vi "AllVIs.vi"   [LabVIEW 2023]
doc: "This VI hosts the full list of Redis in LabVIEW developed VIs."
uses:
  Palette/Redis Commands/Connection/AUTH.vi
  Palette/Redis Commands/Hashes/HSET.vi
  Palette/Redis Commands/Keys/SCAN.vi
  Palette/Redis Commands/Lists/RPUSH.vi
  Palette/Redis Commands/Pub-Sub/PUBLISH.vi
  Palette/Redis Commands/Server/INFO.vi
  Palette/Redis Commands/Sets/SADD.vi
  Palette/Redis Commands/Sorted-Sets/ZADD.vi
  Palette/Redis Commands/Strings/MSET.vi
  Palette/Redis Commands/Transactions/EXEC.vi
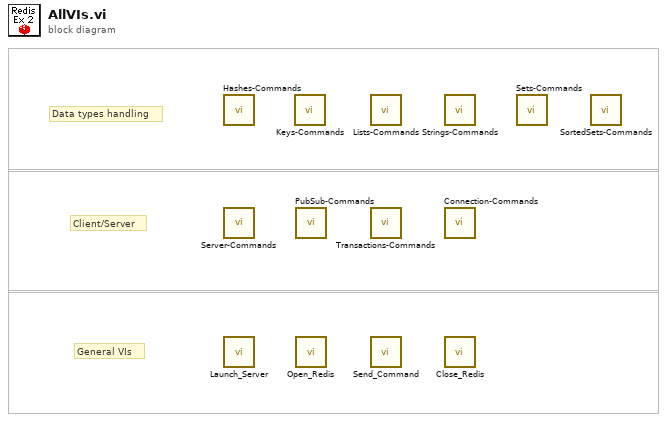
[diagram p0: block diagram]
diagram:
  # "General VIs"
  # "Client/Server"
  # "Data types handling"
  n1 = call-poly "Hashes-Commands.vi"() -> ()  [unwired: 13 in, 3 out]
  n2 = call-poly "Server-Commands.vi"() -> ()  [unwired: 13 in, 3 out]
  n3 = call "Launch_Server.vi"() -> ()  [unwired: 10 in, 2 out]
  n4 = call-poly "Keys-Commands.vi"() -> ()  [unwired: 13 in, 3 out]
  n5 = call-poly "PubSub-Commands.vi"() -> ()  [unwired: 13 in, 3 out]
  n6 = call "Open_Redis.vi"() -> ()  [unwired: 13 in, 3 out]
  n7 = call-poly "Lists-Commands.vi"() -> ()  [unwired: 13 in, 3 out]
  n8 = call-poly "Transactions-Commands.vi"() -> ()  [unwired: 13 in, 3 out]
  n9 = call "Send_Command.vi"() -> ()  [unwired: 8 in, 4 out]
  n10 = call-poly "Strings-Commands.vi"() -> ()  [unwired: 13 in, 3 out]
  n11 = call-poly "Connection-Commands.vi"() -> ()  [unwired: 13 in, 3 out]
  n12 = call "Close_Redis.vi"() -> ()  [unwired: 12 in, 4 out]
  n13 = call-poly "Sets-Commands.vi"() -> ()  [unwired: 13 in, 3 out]
  n14 = call-poly "SortedSets-Commands.vi"() -> ()  [unwired: 13 in, 3 out]
